vi "Labview_simulation_2.vi"() -> ()   [LabVIEW 2021]
uses:
  <vilib>/sound2/lvsound2.llb/Sound Data Format.ctl
  <vilib>/addons/Modulation/Analog/support/mod_Set Error Source.vi
  <vilib>/sound2/lvsound2.llb/Sound File Info (path).vi
  <vilib>/addons/Modulation/Digital/Support/Common/Validators/mod_Generate Filter Coefficients Validate.vi
  <vilib>/addons/Modulation/Digital/General/subVIs/mod_Generate Filter Coefficients.vi
  <vilib>/addons/Modulation/Digital/General/MT Generate PSK System Parameters(M).vi
  <vilib>/addons/Modulation/niDMT.lvlib
  <vilib>/addons/Modulation/niAMT.lvlib
panel:
  out "data":waveform(dbl)[](array[waveform])
  in  "samples per symbol (16)":i32=16
  in  "differential PSK":enum16{"disable", "enable"}(ring)
  out "sound format":T1={"sample rate (S/s)"=22050.0, "number of channels"=2, "bits per sample"=16}
  in  "matched samples per symbol (16)":i32=16
  in  "Path input":path
  out "Constellation Graph":T2(graph)
  in  "pulse shaping samples per symbol (16)":i32=16
  in  "pulse shaping filter (none)":T3(ring)
  out "Q":cluster{"t0":dbl, "dt":dbl, "Y":dbl[]}(graph)
  out "I":cluster{"t0":dbl, "dt":dbl, "Y":dbl[]}(graph)
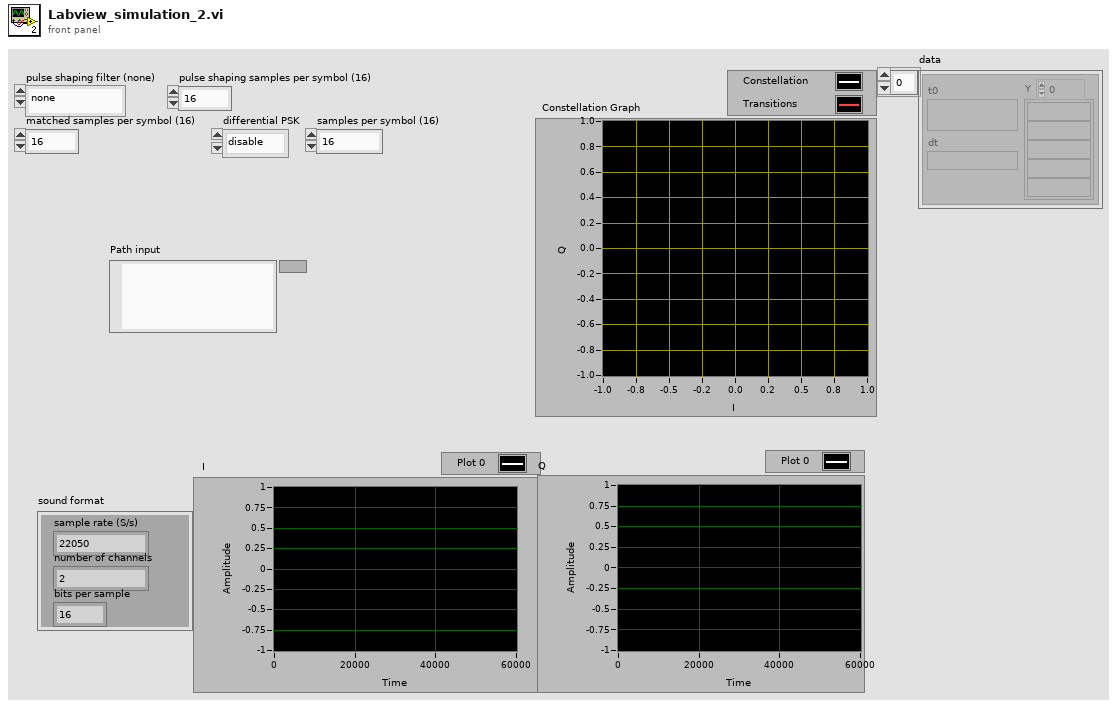
[diagram p1: front panel]
types:
  T1 = typedef "Sound Data Format.ctl" = cluster{"sample rate (S/s)":dbl, "number of channels":i32, "bits per sample":i32}
  T2 = cluster{"Decimated Array":dbl[], "Decimated Array":dbl[]}[]
  T3 = enum16{"none", "Raised Cosine", "Root Raised Cos", "Gaussian"}
  T4 = enum16{"FSK", "PSK", "QAM", "MSK", "PAM", "ASK", "CPM"}
  T5 = cluster{"samples per symbol (16)":i32, "symbol map":cdb[], "differential PSK":enum16{"disable", "enable"}, "PSK type":u16}
  T6 = typedef "niAMT.lvlib/Complex Data Waveform.ctl" = cluster{"t0":dbl, "dt":dbl, "Y":cdb[]}
  T7 = cluster{"constellation":dbl[], "oversampled data":dbl[]}[]
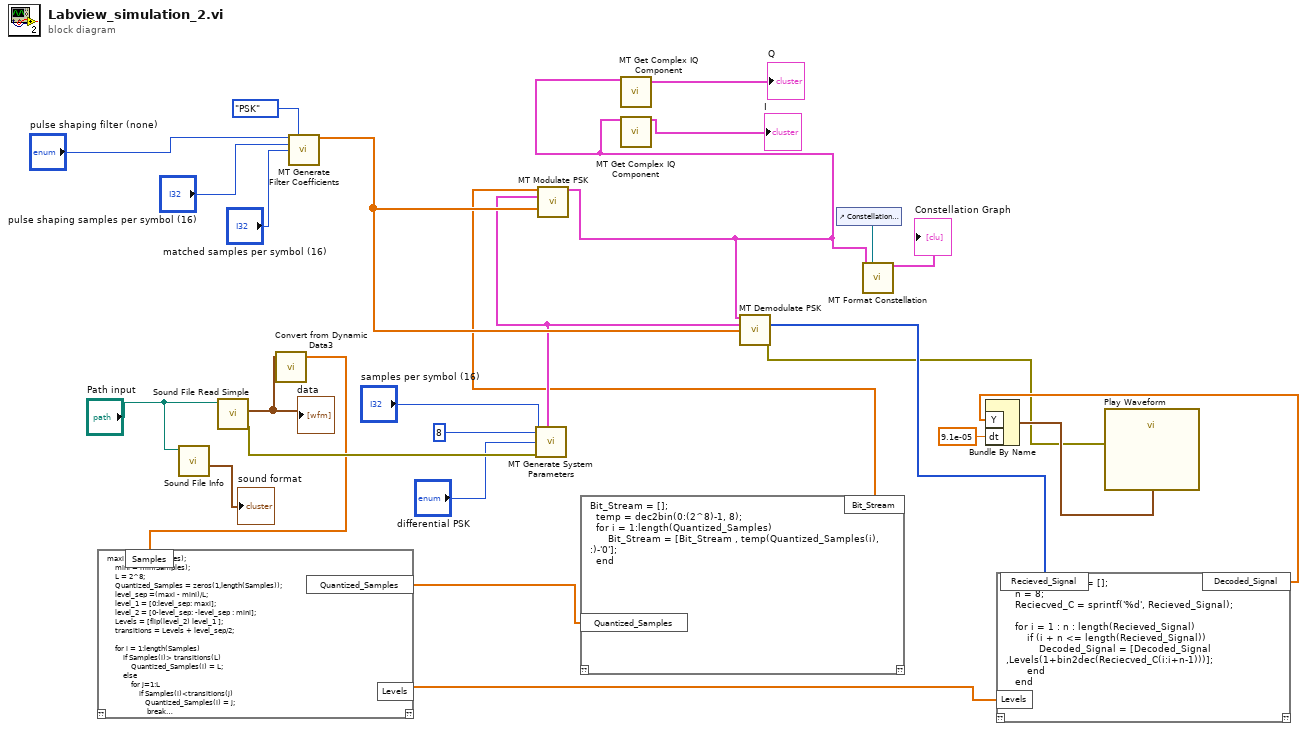
[diagram p0: block diagram]
diagram:
  n1 = call-poly <vilib>:"Sound File Info.vi"("path"="Path input") -> ("sound format"=→"sound format":T1)  [unwired: 7 in, 3 out]
  n2 = call <vilib>:"Sound File Read Simple.vi"("path"="Path input") -> ("error out"=w16:errorcluster, "data"=w6:waveform(dbl)[])  [unwired: 7 in, 2 out]
  "data" <- w6
  n3 = call "Convert from Dynamic Data3"("Dynamic Data Type"=w6) -> ("Array"=w5:dbl[])  [unwired: 3 in]
  n4 = script code="maxi = max(Samples);\n    mini = min(Samples);\n    L = 2^8;\n    Quantized_Samples = zeros(1,length(Samples));\n    level_sep =(maxi - mini)/L; \n    level_1 = [0:level_sep: maxi];\n    level_2 = [0-level_sep: -level_sep : mini];\n    Levels = [flip(level_2) level_1 ];\n    transitions = Levels + level_sep/2;\n    \n    for i = 1:length(Samples)\n        if Samples(i)> transitions(L)\n            Quantized_Samples(i) = L;\n        else\n            for j=1:L\n                if Samples(i)<transitions(j)\n                   Quantized_Samples(i) = j;\n                    break\n                end\n            end\n        end\n    end"("Samples"=w5) -> ("Quantized_Samples"=w9:dbl[], "Levels"=w10:dbl[])  [unwired: 1 in, 1 out]
  n5 = call <vilib>:"MT Generate Filter Coefficients.vi"("pulse shaping filter (none)"="pulse shaping filter (none)", "modulation type"=T4."PSK", "pulse shaping samples per symbol (16)"="pulse shaping samples per symbol (16)", "matched samples per symbol (16)"="matched samples per symbol (16)") -> ("pulse shaping filter coefficients"=w21:dbl[])  [unwired: 9 in, 2 out]
  n6 = call-poly <vilib>:"MT Generate System Parameters.vi"("samples per symbol (16)"="samples per symbol (16)", "M-PSK (4)"=8, "differential PSK"="differential PSK", "error in (no error)"=w16) -> ("PSK system parameters"=w12:T5)  [unwired: 9 in, 2 out]
  n7 = script code="Bit_Stream = [];\n  temp = dec2bin(0:(2^8)-1, 8);  \n  for i = 1:length(Quantized_Samples)\n      Bit_Stream = [Bit_Stream , temp(Quantized_Samples(i), :)-'0'];\n  end"("Quantized_Samples"=w9) -> ("Bit_Stream"=w8:dbl[])  [unwired: 1 in, 1 out]
  n8 = call <vilib>:"MT Modulate PSK.vi"("input bit stream"=w8, "PSK system parameters"=w12, "pulse shaping filter coefficients"=w21) -> ("output complex waveform"=w11:T6)  [unwired: 10 in, 2 out]
  n9 = call <vilib>:"MT Get Complex IQ Component.vi"("IQ data (complex) in"=w11) -> ("IQ data (complex) out"=→"Q":cluster{"t0":dbl, "dt":dbl, "Y":cdb[]})  [unwired: 12 in, 2 out]
  n10 = call <vilib>:"MT Get Complex IQ Component.vi"("IQ data (complex) in"=w11) -> ("IQ data (complex) out"=→"I":cluster{"t0":dbl, "dt":dbl, "Y":cdb[]})  [unwired: 12 in, 2 out]
  n11 = call <vilib>:"MT Demodulate PSK.vi"("input complex waveform"=w11, "PSK system parameters"=w12, "matched filter coefficients"=w21) -> ("output bit stream"=w7:i8[], "error out"=w1:errorcluster)  [unwired: 8 in, 3 out]
  n12 = control-ref of="Constellation Graph"() -> (w23:refnum<vi>)
  n13 = call <vilib>:"MT Format Constellation.vi"("waveform"=w11, "constellation reference"=w23) -> ("constellation graph"=→"Constellation Graph":T7)  [unwired: 3 in, 10 out]
  n14 = script code="Decoded_Signal = [];\n   n = 8;\n   Reciecved_C = sprintf('%d', Recieved_Signal);\n   \n   for i = 1 : n : length(Recieved_Signal)\n       if (i + n <= length(Recieved_Signal))\n           Decoded_Signal = [Decoded_Signal ,Levels(1+bin2dec(Reciecved_C(i:i+n-1)))];\n       end\n   end"("Recieved_Signal"=w7, "Levels"=w10) -> ("Decoded_Signal"=w4:dbl[])  [unwired: 1 in, 1 out]
  n15 = Bundle By Name("Y"=w4, "dt"=9.1e-05) -> (w3:waveform(dbl))  [unwired: 1 in]
  n16 = call "Play Waveform"("Data"=w3, "error in"=w1) -> ()  [unwired: 17 in, 1 out]
